vi "yaw-roll-pitch.vi"() -> ()   [LabVIEW 2014]
uses:
  <vilib>/picture/3D Picture Control/Object/Create Object (name).vi
  <vilib>/picture/3D Picture Control/NI_3D Picture Control.lvlib
panel:
  out "Angle":sgl
  out "Axis":cluster{"X":sgl, "Y":sgl, "Z":sgl}
  in  "Yaw":dbl(knob) scale=0.0..360.0
  in  "Pitch":dbl(knob) scale=0.0..360.0
  in  "Roll":dbl(knob) scale=0.0..360.0
  in  "Stop":bool
  out "3D Picture":refnum<vi>(3d-picture)
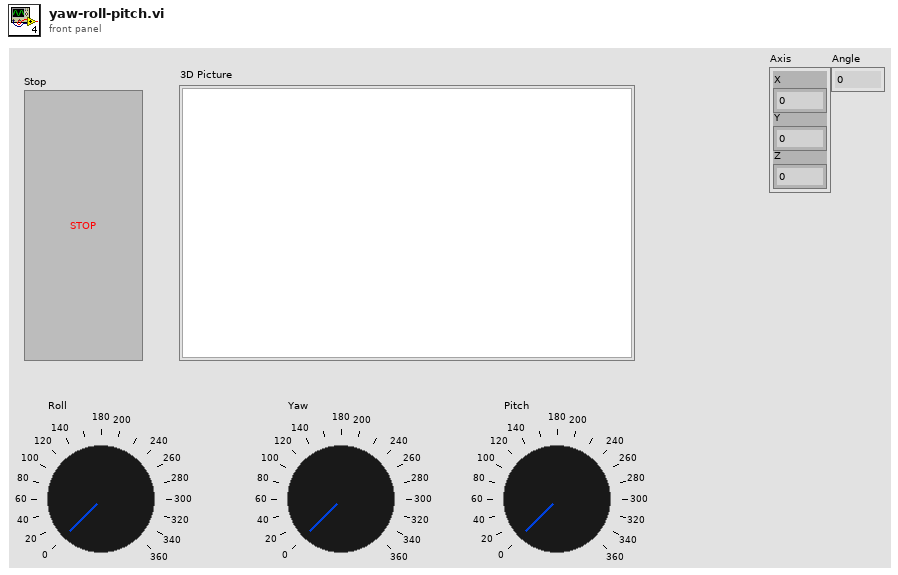
[diagram p1: front panel]
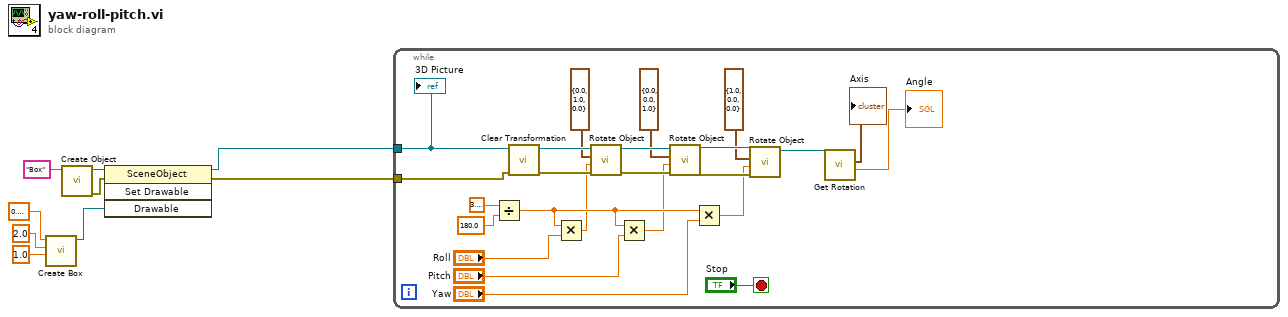
[diagram p0: block diagram]
diagram:
  n1 = call <vilib>:"Create Box.vi"("Length Z"=sgl 1.0, "Length Y"=sgl 2.0, "Length X"=sgl 0.2) -> ("New Box Refnum"=w9:refnum<vi>)  [unwired: 7 in, 1 out]
  n2 = call-poly <vilib>:"Create Object.vi"("Name"="Box") -> ("error out"=w8:errorcluster, "Scene:New Object"=w7:refnum<vi>)  [unwired: 9 in]
  n3 = invoke class="SceneObject" method="Set Drawable"(reference=w7, error in=w8, "Drawable"=w9) -> (reference out=w2:refnum<vi>, error out=w1:errorcluster)  [unwired: 1 in, 2 out]
  n4 = while {
    tunnel: w2 -> [w14]
    tunnel: w1 -> [w13]
    stop <- "Stop" stop-if-true
    n5 = Divide(x=3.141592653589793, y=180.0) -> (x/y=w22:dbl)
    n6 = call <vilib>:"Clear Transformation.vi"("error in (no error)"=w13, "Object Refnum In"=w14) -> ("error out"=w30:errorcluster, "Object Refnum Out"=w31:refnum<vi>)  [unwired: 8 in]
    n7 = Multiply(x=w22, y="Roll") -> (x*y=w19:dbl)
    n8 = call <vilib>:"Rotate Object.vi"("error in (no error)"=w30, "Angle"=w19, "Axis"=cluster{"X":sgl, "Y":sgl, "Z":sgl} {"X"=0.0, "Y"=1.0, "Z"=0.0}, "Scene.Object In"=w31) -> ("error out"=w32:errorcluster, "Scene.Object Out"=w33:refnum<vi>)  [unwired: 6 in]
    n9 = Multiply(x=w22, y="Pitch") -> (x*y=w18:dbl)
    n10 = call <vilib>:"Rotate Object.vi"("error in (no error)"=w32, "Angle"=w18, "Axis"=cluster{"X":sgl, "Y":sgl, "Z":sgl} {"X"=0.0, "Y"=0.0, "Z"=1.0}, "Scene.Object In"=w33) -> ("error out"=w25:errorcluster, "Scene.Object Out"=w26:refnum<vi>)  [unwired: 6 in]
    n11 = Multiply(x=w22, y="Yaw") -> (x*y=w21:dbl)
    n12 = call <vilib>:"Rotate Object.vi"("error in (no error)"=w25, "Angle"=w21, "Axis"=cluster{"X":sgl, "Y":sgl, "Z":sgl} {"X"=1.0, "Y"=0.0, "Z"=0.0}, "Scene.Object In"=w26) -> ("Scene.Object Out"=w12:refnum<vi>)  [unwired: 6 in, 1 out]
    n13 = call <vilib>:"Get Rotation.vi"("Scene Object"=w12) -> ("Angle"=→"Angle":sgl, "Axis"=→"Axis":cluster{"X":sgl, "Y":sgl, "Z":sgl})  [unwired: 7 in, 2 out]
    "3D Picture" <- w14
  }
